vi "BurnInErrorHandler.vi"(5 "FilePathErrors":errorcluster[](array[cluster])) -> ()   [LabVIEW 2012]
uses:
  Constants.vi
panel:
  in  "error in (no error)":errorcluster
  out "error out":errorcluster
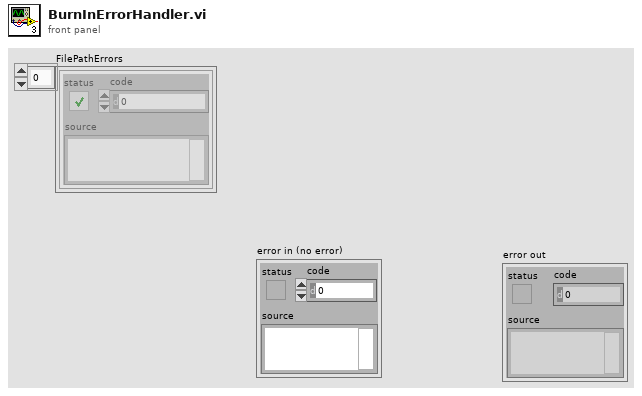
[diagram p1: front panel]
types:
  T1 = typedef "BurnInErrors.ctl" = cluster{"error in (no error)":errorcluster, T2}
  T2 = typedef "ErrorActions.ctl" = enum16{"Shutdown", "Warning", "Reset"}
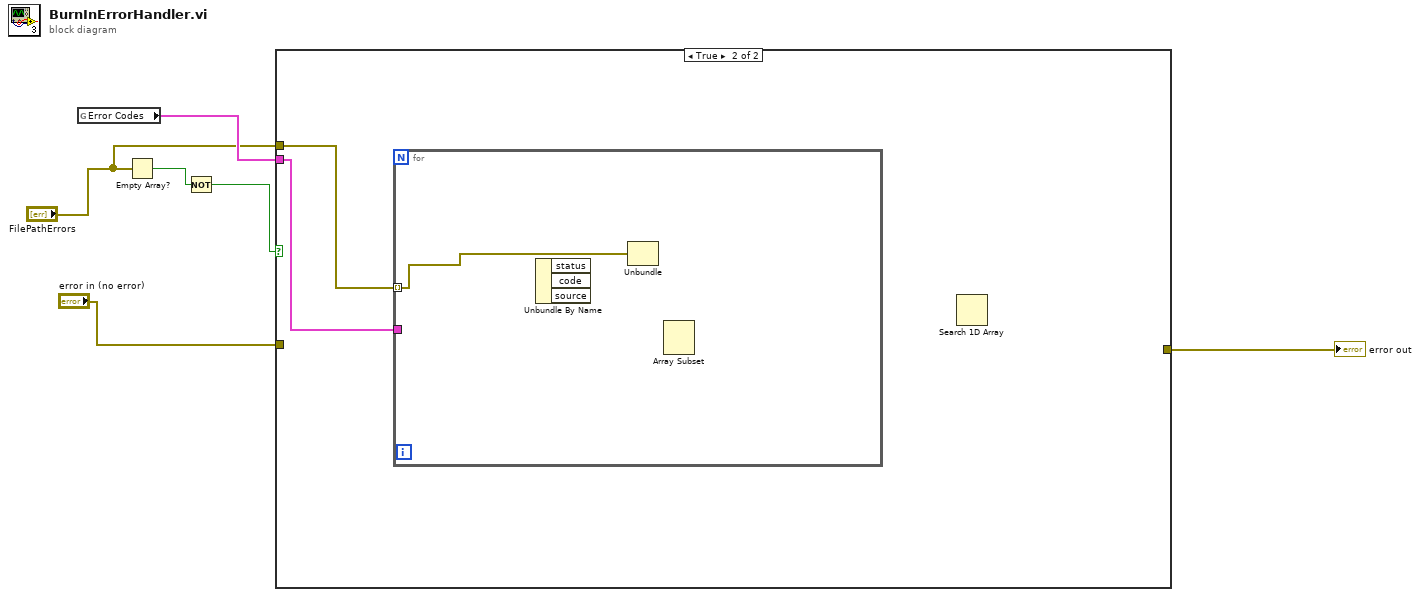
[diagram p0: block diagram]
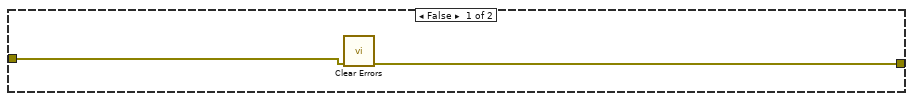
[diagram p2: hidden frame]
diagram:
  n1 = global read "Constants.vi" "Error Codes"() -> (w4:T1[])
  n2 = Empty Array?(array="FilePathErrors") -> (empty?=w6:bool)
  n3 = Not(x=w6) -> (.not. x?=w5:bool)
  n4 = case shown="True" w5 {
    tunnel: w4 -> [_ w9]
    tunnel: "error in (no error)" -> [w8 _]
    tunnel: [w7 _] -> w2
    tunnel: "FilePathErrors" -> [_ w10]
    frame False {
      n5 = call <vilib>:"Clear Errors.vi"("error in (no error)"=w8) -> ("error out"=w7:errorcluster)  [unwired: 6 in]
    }
    frame True {
      n6 = for {
        tunnel: w10 -> [w11] mode=indexing
        tunnel: w9 -> [_]
        n7 = Unbundle By Name() -> ()  [unwired: 1 in, 3 out]
        n8 = Unbundle(w11) -> ()  [unwired: 3 out]
        n9 = Array Subset() -> ()  [unwired: 3 in, 1 out]
      }
      n10 = Search 1D Array() -> ()  [unwired: 3 in, 1 out]
    }
  }
  "error out" <- w2
